vi "Auto Align.vi"() -> (3 "Rotational Velocity":cluster{"output":dbl})   [LabVIEW 2020]
uses:
  <vilib>/Rock Robotics/Network Tables/NT Read Number.vi
panel:
  in  "alpha":dbl=nan format="%.2f"
  out "Output":dbl(graph)
  in  "PID gains":T1={"proportional gain (Kp)"=6.0, "integral time (Ki)"=0.0, "derivative time (Kd)"=0.0} {"derivative time (Kd)" format="%.3f"; "integral time (Ki)" format="%.3f"; "proportional gain (Kp)" format="%.3f"}
  in  "deadband":dbl=1.5 format="%#_13g"
  out "Input":dbl(graph)
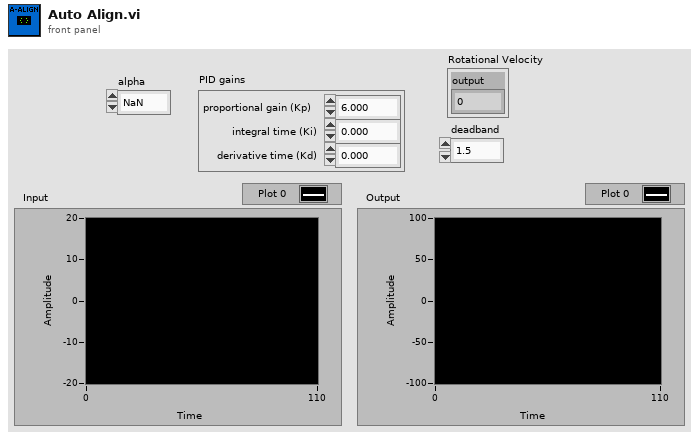
[diagram p1: front panel]
types:
  T1 = cluster{"proportional gain (Kp)":dbl, "integral time (Ki)":dbl, "derivative time (Kd)":dbl}
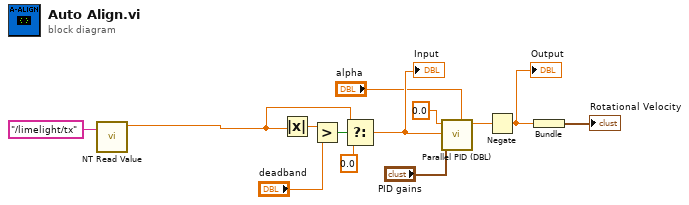
[diagram p0: block diagram]
diagram:
  n1 = call-poly <vilib>:"NT Read Value.vi"("Name"="/limelight/tx") -> ("Numeric"=w1:dbl)  [unwired: 9 in, 1 out]
  n2 = Absolute Value(x=w1) -> (abs(x)=w11:dbl)
  n3 = Greater?(x=w11, y="deadband") -> (0:w9:bool)
  n4 = Select(t=w1, s=w9, f=0.0) -> (s? t:f=w6:dbl)
  "Input" <- w6
  n5 = call <vilib>:"Parallel PID (DBL).vi"("alpha"="alpha", "PID gains"="PID gains", "process variable"=w6, "setpoint"=0.0) -> ("output"=w4:dbl)  [unwired: 4 in, 3 out]
  n6 = Negate(x=w4) -> (-x=w2:dbl)
  "Output" <- w2
  n7 = Bundle(w2) -> (→"Rotational Velocity":cluster{dbl})  [unwired: 1 in]
